vi "G#Interface_Create.vi"(0 "reference in":refnum<class "G#Object.lvclass">, 2 "G#Object in":refnum<class "G#Object.lvclass">, 5 "error in (no error)":errorcluster) -> (14 "reference out":refnum<class "G#Object.lvclass">, 19 "error out":errorcluster)   [LabVIEW 2020, in "G#Object.lvclass"]
doc: "Creates the G#Interface for the G#Object."
uses:
  <vilib>/addons/_AddQ/G#Object/G#Object.lvclass
  <vilib>/addons/_AddQ/G#Object/G#Object.lvclass/G#Object.ctl
panel:
  # "OBSOLETE!\nFor backward compability"
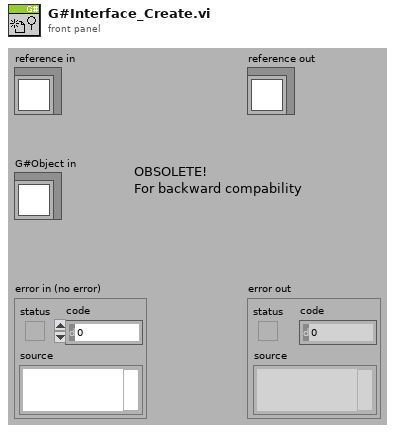
[diagram p1: front panel]
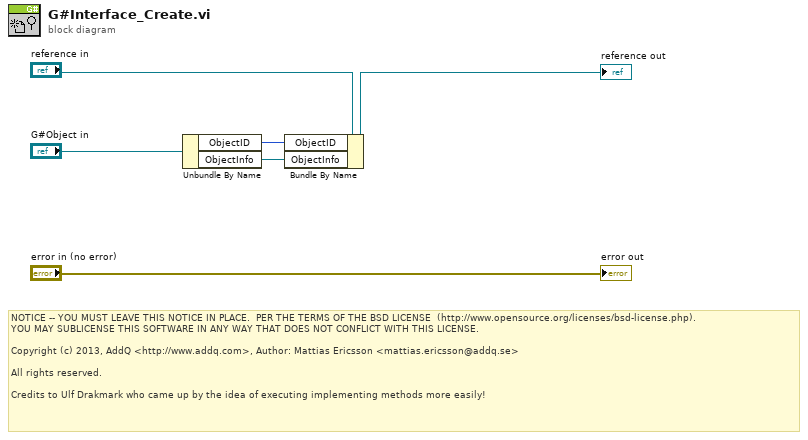
[diagram p0: block diagram]
diagram:
  # "NOTICE -- YOU MUST LEAVE THIS NOTICE IN PLACE.  PER THE TERMS OF THE BSD LICENSE  (http://www.opensource.org/licenses/bsd-license.php).\nYOU MAY SUBLICENSE THIS SOFTWARE IN ANY WAY THAT DOES NOT CONFLICT WITH THIS LICENSE.\n\nCopyright (c) 2013, AddQ <http://www.addq.com>, Author: Mattias Ericsson <mattias.ericsson@addq.se>\n\nAll rights reserved.\n\nCredits to Ulf Drakmark who came up by the idea of executing implementing methods more easily!"
  n1 = Unbundle By Name("G#Object in") -> ("ObjectID"=w2:u32, "ObjectInfo"=w1:refnum<queue>)
  n2 = Bundle By Name(cluster="reference in", "ObjectID"=w2, "ObjectInfo"=w1) -> (→"reference out":refnum<class "G#Object.lvclass">)
  "error out" <- "error in (no error)"
